vi "Autonomous Independent.vi"   [LabVIEW 2017] (continued)
                  n1161 = call <vilib>:"WPI_RobotDriveTankDrive.vi"("Right axis value"=w3971, "Left axis value"=w3971, "RobotDriveDevRef"=w3970) -> ("RobotDriveDevRef"=w3969:T1)  [unwired: 6 in, 2 out]
                  n1162 = global write "Robot Global Data.vi" "Axes"(w3975) -> ()
                }
                frame #5 {
                  n1163 = global write "Robot Global Data.vi" "Current State"(FALSE ("Current State")) -> ()
                  n1164 = Wait (ms)(milliseconds to wait=u32 400) -> ()  [unwired: 1 out]
                }
                frame #6 {
                  n1165 = global read "Robot Global Data.vi" "Axes"() -> (w3989:dbl[])
                  n1166 = Array To Cluster(array=w3989) -> (cluster=w3988:T15)
                  n1167 = Bundle By Name(cluster=w3988, "Axes[1]"=-1.0) -> (w3991:T15)
                  n1168 = Cluster To Array(cluster=w3991) -> (array=w3990:dbl[])
                  n1169 = global write "Robot Global Data.vi" "Axes"(w3990) -> ()
                }
                frame #7 {
                  n1170 = call "PID Distance.vi"("Distance"=7.0, "Angle"=90.0, "RightEncoder"=w3996, "LeftEncoder"=w3997, "GyroDevRef"=w4002, "RobotDriveDevRef"=w4001) -> ("RightEncoder 2"=w3993:T11, "LeftEncoder 2"=w3994:T11, "GyroDevRef 2"=w3995:T8, "RobotDriveDevRef 2"=w4000:T1)  [unwired: 2 in]
                }
                frame #8 {
                  n1171 = global write "Robot Global Data.vi" "Lift_Position"(1.0) -> ()
                  n1172 = call "PID turning.vi"("Angle"=155.0, "GyroDevRef"=w4008, "RobotDriveDevRef"=w4009) -> ("GyroDevRef 2"=w4004:T8, "RobotDriveDevRef 2"=w4005:T1)  [unwired: 7 in]
                }
                frame #9 {
                  n1173 = global read "Robot Global Data.vi" "PIXY Output"() -> (w4022:T16)
                  n1174 = Unbundle By Name(w4022) -> ("SIGNATURE NUMBER"=w4021:u16)
                  n1175 = global read "Robot Global Data.vi" "Cube Signature"() -> (w4020:dbl)
                  n1176 = Equal?(x=w4021, y=w4020) -> (x = y?=w4019:bool)
                  n1177 = case shown="False" w4019 {
                    tunnel: [w4029 w4033] -> w4011
                    tunnel: [w4028 w4034] -> w4012
                    tunnel: [w4027 w4035] -> w4013
                    tunnel: [w4031 w4036] -> w4014
                    tunnel: w4016 -> [w4028 w4034]
                    tunnel: w4015 -> [w4029 w4033]
                    tunnel: w4017 -> [w4030 w4035]
                    tunnel: w4018 -> [w4032 w4036]
                    frame True {
                      n1178 = call <vilib>:"WPI_GyroGetAngle.vi"("GyroDevRef"=w4030) -> ("Angle"=w4026:dbl, "GyroDevRef"=w4027:T8)  [unwired: 6 in, 3 out]
                      n1179 = In Range and Coerce(upper limit=170.0, x=w4026, lower limit=155.0) -> (coerced(x)=w4025:dbl)  [unwired: 1 out]
                      n1180 = global write "Robot Global Data.vi" "Tracked Angle"(w4025) -> ()
                      n1181 = call "PID vision.vi"("RobotDriveDevRef in"=w4032) -> ("RobotDriveDevRef out"=w4031:T1)  [unwired: 9 in, 1 out]
                    }
                    frame False {
                      n1182 = global write "Robot Global Data.vi" "Tracked Angle"(155.0) -> ()
                    }
                  }
                }
                frame #10 {
                  n1183 = call <vilib>:"WPI_EncoderReset.vi"("EncoderDevRef"=w4044) -> ("EncoderDevRef"=w4039:T11)  [unwired: 9 in, 1 out]
                  n1184 = Wait (ms)(milliseconds to wait=u32 10) -> ()  [unwired: 1 out]
                  n1185 = call <vilib>:"WPI_EncoderReset.vi"("EncoderDevRef"=w4043) -> ("EncoderDevRef"=w4038:T11)  [unwired: 9 in, 1 out]
                }
                frame #11 {
                  n1186 = global write "Robot Global Data.vi" "Lift_Position"(0.0) -> ()
                  n1187 = global read "Robot Global Data.vi" "Axes"() -> (w4059:dbl[])
                  n1188 = Array To Cluster(array=w4059) -> (cluster=w4058:T15)
                  n1189 = global read "Robot Global Data.vi" "Tracked Angle"() -> (w4051:dbl)
                  n1190 = Bundle By Name(cluster=w4058, "Axes[1]"=1.0) -> (w4061:T15)
                  n1191 = call "PID with Infrared.vi"("RobotDriveDevRef"=w4055, "Angle"=w4051, "Encoder Limit"=120.0, "GyroDevRef"=w4053, "Left Encoder"=w4048, "Right Encoder"=w4046, "DigitalInputDevRef"=w4050) -> ("RobotDriveDevRef 2"=w4054:T1, "GyroDevRef 2"=w4052:T8, "Left Encoder 2"=w4047:T11, "Right Encoder 2"=w4045:T11)  [unwired: 4 in, 1 out]
                  n1192 = Cluster To Array(cluster=w4061) -> (array=w4060:dbl[])
                  n1193 = global write "Robot Global Data.vi" "Axes"(w4060) -> ()
                }
                frame #12 {
                  n1194 = global write "Robot Global Data.vi" "Current State"(TRUE ("Current State")) -> ()
                  n1195 = Wait (ms)(milliseconds to wait=u32 750) -> ()  [unwired: 1 out]
                }
                frame #13 {
                  n1196 = case shown="\"R\"" w4068 {
                    tunnel: w4072 -> [w4079 w4143 _]
                    tunnel: w4071 -> [w4074 w4142 _]
                    tunnel: w4070 -> [w4078 w4141 _]
                    tunnel: w4069 -> [w4076 w4140 _]
                    frame "L" {
                      n1197 = flat-sequence {
                        tunnel: [w4084] -> w4077
                        tunnel: w4076 -> [w4083]
                        tunnel: [w4082] -> w4075
                        tunnel: w4074 -> [w4081]
                        tunnel: [w4080] -> w4073
                        tunnel: w4079 -> [w4103]
                        tunnel: w4078 -> [w4102]
                        tunnel: w4077 -> [w4098]
                        tunnel: w4075 -> [w4097]
                        tunnel: w4073 -> [w4096]
                        frame #0 {
                          n1198 = global read "Robot Global Data.vi" "Axes"() -> (w4093:dbl[])
                          n1199 = global write "Robot Global Data.vi" "Lift_Position"(2.0) -> ()
                          n1200 = Wait (ms)(milliseconds to wait=u32 250) -> ()  [unwired: 1 out]
                          n1201 = Array To Cluster(array=w4093) -> (cluster=w4092:T15)
                          n1202 = Bundle By Name(cluster=w4092, "Axes[1]"=-1.0) -> (w4095:T15)
                          n1203 = call <vilib>:"WPI_EncoderGet.vi"("EncoderDevRef"=w4083) -> ("Distance"=w4087:dbl, "EncoderDevRef"=w4082:T11)  [unwired: 5 in, 4 out]
                          n1204 = call <vilib>:"WPI_EncoderGet.vi"("EncoderDevRef"=w4081) -> ("Distance"=w4088:dbl, "EncoderDevRef"=w4080:T11)  [unwired: 5 in, 4 out]
                          n1205 = Add(x=w4087, y=w4088) -> (x+y=w4086:dbl)
                          n1206 = Cluster To Array(cluster=w4095) -> (array=w4094:dbl[])
                          n1207 = global write "Robot Global Data.vi" "Axes"(w4094) -> ()
                          n1208 = Divide(x=w4086, y=2.0) -> (x/y=w4084:dbl)
                        }
                        frame #1 {
                          n1209 = Add(x=w4098, y=15.0 ("Distance")) -> (x+y=w4099:dbl)
                          n1210 = global read "Robot Global Data.vi" "Tracked Angle"() -> (w4101:dbl)
                          n1211 = call "PID Distance.vi"("Distance"=w4099, "Angle"=w4101, "RightEncoder"=w4096, "LeftEncoder"=w4097, "GyroDevRef"=w4102, "RobotDriveDevRef"=w4103) -> ()  [unwired: 2 in, 4 out]
                        }
                        frame #2 {
                          n1212 = global read "Robot Global Data.vi" "Axes"() -> (w4107:dbl[])
                          n1213 = Wait (ms)(milliseconds to wait=u32 200) -> ()  [unwired: 1 out]
                          n1214 = Array To Cluster(array=w4107) -> (cluster=w4106:T15)
                          n1215 = Bundle By Name(cluster=w4106, "Axes[1]"=0.5) -> (w4109:T15)
                          n1216 = Cluster To Array(cluster=w4109) -> (array=w4108:dbl[])
                          n1217 = global write "Robot Global Data.vi" "Axes"(w4108) -> ()
                        }
                        frame #3 {
                          n1218 = global write "Robot Global Data.vi" "Current State"(FALSE ("Current State")) -> ()
                          n1219 = Wait (ms)(milliseconds to wait=u32 500) -> ()  [unwired: 1 out]
                        }
                      }
                    }
                    frame "R" {
                      n1220 = flat-sequence {
                        tunnel: w4143 -> [w4154]
                        tunnel: w4142 -> [w4159]
                        tunnel: w4141 -> [w4153]
                        tunnel: w4140 -> [w4152]
                        tunnel: [w4158] -> w4139
                        tunnel: [w4157] -> w4138
                        tunnel: [w4156] -> w4136
                        tunnel: [w4155] -> w4134
                        tunnel: w4139 -> [w4167]
                        tunnel: w4138 -> [w4166]
                        tunnel: [w4165] -> w4137
                        tunnel: w4136 -> [w4165]
                        tunnel: [w4164] -> w4135
                        tunnel: w4134 -> [w4164]
                        tunnel: [w4163] -> w4132
                        tunnel: [w4162] -> w4130
                        tunnel: w4137 -> [w4174]
                        tunnel: w4135 -> [w4173]
                        tunnel: [w4172] -> w4133
                        tunnel: w4132 -> [w4172]
                        tunnel: [w4171] -> w4131
                        tunnel: w4130 -> [w4171]
                        tunnel: [w4170] -> w4129
                        tunnel: [w4169] -> w4128
                        tunnel: w4133 -> [w4184]
                        tunnel: w4131 -> [w4183]
                        tunnel: w4129 -> [w4182]
                        tunnel: w4128 -> [w4181]
                        tunnel: [w4180] -> w4127
                        tunnel: [w4179] -> w4126
                        tunnel: [w4177] -> w4125
                        tunnel: [w4176] -> w4124
                        tunnel: [w4190] -> w4123
                        tunnel: [w4189] -> w4122
                        tunnel: [w4188] -> w4121
                        tunnel: [w4187] -> w4120
                        tunnel: w4124 -> [w4187]
                        tunnel: w4125 -> [w4188]
                        tunnel: w4126 -> [w4189]
                        tunnel: w4127 -> [w4190]
                        tunnel: [w4200] -> w4113
                        tunnel: w4123 -> [w4200]
                        tunnel: [w4199] -> w4115
                        tunnel: w4122 -> [w4199]
                        tunnel: [w4198] -> w4117
                        tunnel: w4121 -> [w4198]
                        tunnel: [w4197] -> w4119
                        tunnel: w4120 -> [w4197]
                        tunnel: w4119 -> [w4212]
                        tunnel: [w4212] -> w4118
                        tunnel: w4117 -> [w4211]
                        tunnel: [w4211] -> w4116
                        tunnel: w4115 -> [w4210]
                        tunnel: [w4210] -> w4114
                        tunnel: w4113 -> [w4209]
                        tunnel: [w4209] -> w4112
                        tunnel: w4118 -> [w4213]
                        tunnel: w4116 -> [w4214]
                        tunnel: w4114 -> [w4215]
                        tunnel: w4112 -> [w4216]
                        frame #0 {
                          n1221 = global read "Robot Global Data.vi" "Axes"() -> (w4148:dbl[])
                          n1222 = global write "Robot Global Data.vi" "Lift_Position"(2.0) -> ()
                          n1223 = Wait (ms)(milliseconds to wait=u32 250) -> ()  [unwired: 1 out]
                          n1224 = Array To Cluster(array=w4148) -> (cluster=w4147:T15)
                          n1225 = Bundle By Name(cluster=w4147, "Axes[1]"=-1.0) -> (w4150:T15)
                          n1226 = Cluster To Array(cluster=w4150) -> (array=w4149:dbl[])
                          n1227 = global write "Robot Global Data.vi" "Axes"(w4149) -> ()
                        }
                        frame #1 {
                          n1228 = global read "Robot Global Data.vi" "Tracked Angle"() -> (w4151:dbl)
                          n1229 = call "PID Distance.vi"("Distance"=-10.0, "Angle"=w4151, "RightEncoder"=w4159, "LeftEncoder"=w4152, "GyroDevRef"=w4153, "RobotDriveDevRef"=w4154) -> ("RightEncoder 2"=w4155:T11, "LeftEncoder 2"=w4156:T11, "GyroDevRef 2"=w4157:T8, "RobotDriveDevRef 2"=w4158:T1)  [unwired: 2 in]
                        }
                        frame #2 {
                          n1230 = call "PID turning.vi"("Angle"=90.0, "GyroDevRef"=w4166, "RobotDriveDevRef"=w4167) -> ("GyroDevRef 2"=w4162:T8, "RobotDriveDevRef 2"=w4163:T1)  [unwired: 7 in]
                          n1231 = global write "Robot Global Data.vi" "Lift_Position"(3.0) -> ()
                        }
                        frame #3 {
                          n1232 = call <vilib>:"WPI_EncoderReset.vi"("EncoderDevRef"=w4174) -> ("EncoderDevRef"=w4170:T11)  [unwired: 9 in, 1 out]
                          n1233 = Wait (ms)(milliseconds to wait=u32 10) -> ()  [unwired: 1 out]
                          n1234 = call <vilib>:"WPI_EncoderReset.vi"("EncoderDevRef"=w4173) -> ("EncoderDevRef"=w4169:T11)  [unwired: 9 in, 1 out]
                        }
                        frame #4 {
                          n1235 = call "PID Distance.vi"("Distance"=30.0, "Angle"=90.0, "RightEncoder"=w4181, "LeftEncoder"=w4182, "GyroDevRef"=w4183, "RobotDriveDevRef"=w4184) -> ("RightEncoder 2"=w4176:T11, "LeftEncoder 2"=w4177:T11, "GyroDevRef 2"=w4179:T8, "RobotDriveDevRef 2"=w4180:T1)  [unwired: 2 in]
                          n1236 = global write "Robot Global Data.vi" "Lift_Position"(3.0) -> ()
                        }
                        frame #5 {
                          n1237 = global read "Robot Global Data.vi" "Axes"() -> (w4194:dbl[])
                          n1238 = Wait (ms)(milliseconds to wait=u32 500) -> ()  [unwired: 1 out]
                          n1239 = Array To Cluster(array=w4194) -> (cluster=w4193:T15)
                          n1240 = Bundle By Name(cluster=w4193, "Axes[1]"=0.3) -> (w4196:T15)
                          n1241 = Cluster To Array(cluster=w4196) -> (array=w4195:dbl[])
                          n1242 = global write "Robot Global Data.vi" "Axes"(w4195) -> ()
                        }
                        frame #6 {
                          n1243 = global write "Robot Global Data.vi" "Current State"(FALSE ("Current State")) -> ()
                          n1244 = Wait (ms)(milliseconds to wait=u32 400) -> ()  [unwired: 1 out]
                        }
                        frame #7 {
                          n1245 = global read "Robot Global Data.vi" "Axes"() -> (w4206:dbl[])
                          n1246 = Wait (ms)(milliseconds to wait=u32 250) -> ()  [unwired: 1 out]
                          n1247 = Array To Cluster(array=w4206) -> (cluster=w4205:T15)
                          n1248 = Bundle By Name(cluster=w4205, "Axes[1]"=-1.0) -> (w4208:T15)
                          n1249 = Cluster To Array(cluster=w4208) -> (array=w4207:dbl[])
                          n1250 = global write "Robot Global Data.vi" "Axes"(w4207) -> ()
                        }
                        frame #8 {
                          n1251 = call "PID Distance.vi"("Distance"=10.0, "Angle"=90.0, "RightEncoder"=w4213, "LeftEncoder"=w4214, "GyroDevRef"=w4215, "RobotDriveDevRef"=w4216) -> ()  [unwired: 2 in, 4 out]
                        }
                        frame #9 {
                          n1252 = global write "Robot Global Data.vi" "Lift_Position"(1.0) -> ()
                        }
                      }
                    }
                    frame Default {
                    }
                  }
                }
              }
            }
            frame Default {
              n1253 = flat-sequence {
                tunnel: w4221 -> [w4229]
                tunnel: w4220 -> [w4228]
                tunnel: w4222 -> [w4226]
                tunnel: [w4227] -> w4224
                tunnel: w4223 -> [w4225]
                tunnel: w4224 -> [w4232]
                frame #0 {
                  n1254 = call "PID Distance.vi"("Distance"=90.0, "Angle"=0.0, "RightEncoder"=w4225, "LeftEncoder"=w4226, "GyroDevRef"=w4228, "RobotDriveDevRef"=w4229) -> ("RobotDriveDevRef 2"=w4227:T1)  [unwired: 2 in, 3 out]
                }
                frame #1 {
                  w4233 = 0.0
                  n1255 = call <vilib>:"WPI_RobotDriveTankDrive.vi"("Right axis value"=w4233, "Left axis value"=w4233, "RobotDriveDevRef"=w4232) -> ()  [unwired: 6 in, 3 out]
                }
              }
            }
          }
        }
      }
    }
    frame "Left Switch" {
      n1256 = flat-sequence {
        tunnel: w4237 -> [w4256]
        tunnel: w4238 -> [w4262]
        tunnel: w4239 -> [w4261]
        tunnel: [w4260] -> w4243
        tunnel: [w4259] -> w4242
        tunnel: [w4258] -> w4241
        tunnel: [w4257] -> w4240
        tunnel: w4236 -> [w4255]
        tunnel: w4234 -> [w4248]
        tunnel: w4243 -> [w4268]
        tunnel: w4242 -> [w4267]
        tunnel: w4241 -> [w4266]
        tunnel: w4240 -> [w4265]
        tunnel: w4235 -> [w4264]
        frame #0 {
          w4263 = 0.0 ("Left axis value")
          n1257 = global write "Robot Global Data.vi" "Lift_Position"(0.0) -> ()
          n1258 = Multiply(x=w4248, y=1000.0) -> (x*y=w4249:dbl)
          n1259 = global write "Robot Global Data.vi" "Current State"(TRUE ("Current State")) -> ()
          n1260 = global write "Robot Global Data.vi" "Raise_Mast"(FALSE ("Current State")) -> ()
          n1261 = Wait (ms)(milliseconds to wait=10) -> ()  [unwired: 1 out]
          n1262 = Less Or Equal?(x=w4249, y=0.0) -> (x <= y?=w4252:bool)
          n1263 = Greater?(x=w4249, y=11000.0) -> (0:w4251:bool)
          n1264 = call <vilib>:"WPI_EncoderReset.vi"("EncoderDevRef"=w4262) -> ("EncoderDevRef"=w4258:T11)  [unwired: 9 in, 1 out]
          n1265 = call <vilib>:"WPI_EncoderReset.vi"("EncoderDevRef"=w4256) -> ("EncoderDevRef"=w4259:T11)  [unwired: 9 in, 1 out]
          n1266 = Or(x=w4251, y=w4252) -> ()  [unwired: 1 out]
          n1267 = call <vilib>:"WPI_GyroReset.vi"("GyroDevRef"=w4261) -> ("GyroDevRef"=w4257:T8)  [unwired: 9 in, 1 out]
          n1268 = call <vilib>:"WPI_RobotDriveTankDrive.vi"("Right axis value"=w4263, "Left axis value"=w4263, "RobotDriveDevRef"=w4255) -> ("RobotDriveDevRef"=w4260:T1)  [unwired: 6 in, 2 out]
        }
        frame #1 {
          n1269 = case shown="\"L\"" w4264 {
            tunnel: w4268 -> [w4280 w4366 w4488]
            tunnel: w4267 -> [w4277 w4363 w4485]
            tunnel: w4266 -> [w4278 w4364 w4486]
            tunnel: w4265 -> [w4279 w4365 w4487]
            frame "L" {
              n1270 = flat-sequence {
                tunnel: w4280 -> [w4297]
                tunnel: w4277 -> [w4295]
                tunnel: w4278 -> [w4296]
                tunnel: w4279 -> [w4298]
                tunnel: [w4293] -> w4276
                tunnel: [w4292] -> w4274
                tunnel: [w4291] -> w4272
                tunnel: [w4290] -> w4270
                tunnel: w4276 -> [w4308]
                tunnel: [w4304] -> w4275
                tunnel: w4274 -> [w4307]
                tunnel: [w4303] -> w4273
                tunnel: w4272 -> [w4306]
                tunnel: [w4302] -> w4271
                tunnel: w4270 -> [w4305]
                tunnel: [w4301] -> w4269
                tunnel: w4275 -> [w4318]
                tunnel: w4273 -> [w4317]
                tunnel: [w4316] -> w4289
                tunnel: [w4315] -> w4288
                tunnel: [w4314] -> w4287
                tunnel: w4271 -> [w4314]
                tunnel: [w4313] -> w4286
                tunnel: w4269 -> [w4313]
                tunnel: w4289 -> [w4329]
                tunnel: [w4328] -> w4285
                tunnel: w4288 -> [w4334]
                tunnel: [w4334] -> w4284
                tunnel: w4287 -> [w4333]
                tunnel: [w4331] -> w4283
                tunnel: w4286 -> [w4332]
                tunnel: [w4330] -> w4282
                tunnel: w4285 -> [w4339]
                tunnel: [w4338] -> w4281
                tunnel: w4284 -> [w4337]
                tunnel: w4283 -> [w4336]
                tunnel: w4282 -> [w4335]
                tunnel: w4281 -> [w4349]
                frame #0 {
                  n1271 = global write "Robot Global Data.vi" "Raise_Mast"(TRUE ("Current State")) -> ()
                  n1272 = call "PID Distance.vi"("Distance"=60.0, "Angle"=0.0, "RightEncoder"=w4295, "LeftEncoder"=w4296, "GyroDevRef"=w4298, "RobotDriveDevRef"=w4297) -> ("RightEncoder 2"=w4290:T11, "LeftEncoder 2"=w4291:T11, "GyroDevRef 2"=w4292:T8, "RobotDriveDevRef 2"=w4293:T1)  [unwired: 2 in]
                }
                frame #1 {
                  n1273 = global write "Robot Global Data.vi" "Lift_Position"(2.0) -> ()
                  n1274 = call "PID Distance.vi"("Distance"=140.0, "Angle"=0.0, "RightEncoder"=w4305, "LeftEncoder"=w4306, "GyroDevRef"=w4307, "RobotDriveDevRef"=w4308) -> ("RightEncoder 2"=w4301:T11, "LeftEncoder 2"=w4302:T11, "GyroDevRef 2"=w4303:T8, "RobotDriveDevRef 2"=w4304:T1)  [unwired: 2 in]
                  n1275 = Wait (ms)(milliseconds to wait=u32 50) -> ()  [unwired: 1 out]
                }
                frame #2 {
                  n1276 = global read "Robot Global Data.vi" "Axes"() -> (w4321:dbl[])
                  n1277 = call "PID turning.vi"("Angle"=90.0, "GyroDevRef"=w4317, "RobotDriveDevRef"=w4318) -> ("GyroDevRef 2"=w4315:T8, "RobotDriveDevRef 2"=w4316:T1)  [unwired: 7 in]
                  n1278 = global write "Robot Global Data.vi" "Lift_Position"(2.0) -> ()
                  n1279 = Array To Cluster(array=w4321) -> (cluster=w4320:T15)
                  n1280 = Bundle By Name(cluster=w4320, "Axes[1]"=-1.0) -> (w4323:T15)
                  n1281 = Cluster To Array(cluster=w4323) -> (array=w4322:dbl[])
                  n1282 = global write "Robot Global Data.vi" "Axes"(w4322) -> ()
                }
                frame #3 {
                  w4327 = 0.0 ("Left axis value")
                  n1283 = call <vilib>:"WPI_EncoderReset.vi"("EncoderDevRef"=w4333) -> ("EncoderDevRef"=w4331:T11)  [unwired: 9 in, 1 out]
                  n1284 = call <vilib>:"WPI_RobotDriveTankDrive.vi"("Right axis value"=w4327, "Left axis value"=w4327, "RobotDriveDevRef"=w4329) -> ("RobotDriveDevRef"=w4328:T1)  [unwired: 6 in, 2 out]
                  n1285 = Wait (ms)(milliseconds to wait=u32 10) -> ()  [unwired: 1 out]
                  n1286 = call <vilib>:"WPI_EncoderReset.vi"("EncoderDevRef"=w4332) -> ("EncoderDevRef"=w4330:T11)  [unwired: 9 in, 1 out]
                }
                frame #4 {
                  n1287 = call "PID Distance.vi"("Distance"=18.0, "Angle"=90.0, "RightEncoder"=w4335, "LeftEncoder"=w4336, "GyroDevRef"=w4337, "RobotDriveDevRef"=w4339) -> ("RobotDriveDevRef 2"=w4338:T1)  [unwired: 2 in, 3 out]
                }
                frame #5 {
                  w4348 = 0.0 ("Left axis value")
                  n1288 = global read "Robot Global Data.vi" "Axes"() -> (w4344:dbl[])
                  n1289 = call <vilib>:"WPI_RobotDriveTankDrive.vi"("Right axis value"=w4348, "Left axis value"=w4348, "RobotDriveDevRef"=w4349) -> ()  [unwired: 6 in, 3 out]
                  n1290 = Wait (ms)(milliseconds to wait=u32 20) -> ()  [unwired: 1 out]
                  n1291 = Array To Cluster(array=w4344) -> (cluster=w4343:T15)
                  n1292 = Bundle By Name(cluster=w4343, "Axes[1]"=-1.0) -> (w4346:T15)
                  n1293 = Cluster To Array(cluster=w4346) -> (array=w4345:dbl[])
                  n1294 = global write "Robot Global Data.vi" "Axes"(w4345) -> ()
                }
                frame #6 {
                  n1295 = global read "Robot Global Data.vi" "Axes"() -> (w4352:dbl[])
                  n1296 = Wait (ms)(milliseconds to wait=u32 500) -> ()  [unwired: 1 out]
                  n1297 = Array To Cluster(array=w4352) -> (cluster=w4351:T15)
                  n1298 = Bundle By Name(cluster=w4351, "Axes[1]"=1.0) -> (w4354:T15)
                  n1299 = Cluster To Array(cluster=w4354) -> (array=w4353:dbl[])
                  n1300 = global write "Robot Global Data.vi" "Axes"(w4353) -> ()
                }
                frame #7 {
                  n1301 = global write "Robot Global Data.vi" "Current State"(FALSE ("Current State")) -> ()
                  n1302 = Wait (ms)(milliseconds to wait=u32 500) -> ()  [unwired: 1 out]
                }
                frame #8 {
                  n1303 = global read "Robot Global Data.vi" "Axes"() -> (w4359:dbl[])
                  n1304 = Array To Cluster(array=w4359) -> (cluster=w4358:T15)
                  n1305 = Bundle By Name(cluster=w4358, "Axes[1]"=-1.0) -> (w4361:T15)
                  n1306 = Cluster To Array(cluster=w4361) -> (array=w4360:dbl[])
                  n1307 = global write "Robot Global Data.vi" "Axes"(w4360) -> ()
                }
              }
            }
            frame "R" {
              n1308 = flat-sequence {
                tunnel: w4365 -> [w4400]
                tunnel: w4364 -> [w4401]
                tunnel: w4363 -> [w4402]
                tunnel: w4366 -> [w4403]
                tunnel: [w4403] -> w4399
                tunnel: [w4402] -> w4398
                tunnel: [w4401] -> w4397
                tunnel: [w4400] -> w4396
                tunnel: [w4406] -> w4395
                tunnel: [w4407] -> w4394
                tunnel: [w4404] -> w4393
                tunnel: [w4405] -> w4392
                tunnel: w4399 -> [w4410]
                tunnel: w4398 -> [w4408]
                tunnel: w4397 -> [w4409]
                tunnel: w4396 -> [w4411]
                tunnel: w4395 -> [w4418]
                tunnel: w4394 -> [w4417]
                tunnel: [w4421] -> w4391
                tunnel: w4393 -> [w4421]
                tunnel: [w4420] -> w4390
                tunnel: w4392 -> [w4420]
                tunnel: [w4416] -> w4389
                tunnel: [w4415] -> w4388
                tunnel: w4391 -> [w4428]
                tunnel: w4390 -> [w4427]
                tunnel: [w4426] -> w4387
                tunnel: [w4425] -> w4386
                tunnel: [w4424] -> w4385
                tunnel: w4389 -> [w4424]
                tunnel: [w4422] -> w4384
                tunnel: w4388 -> [w4422]
                tunnel: w4387 -> [w4432]
                tunnel: w4386 -> [w4433]
                tunnel: w4385 -> [w4437]
                tunnel: w4384 -> [w4436]
                tunnel: [w4435] -> w4383
                tunnel: [w4434] -> w4382
                tunnel: [w4431] -> w4381
                tunnel: [w4430] -> w4380
                tunnel: [w4448] -> w4379
                tunnel: w4383 -> [w4449]
                tunnel: w4382 -> [w4450]
                tunnel: [w4447] -> w4378
                tunnel: [w4446] -> w4377
                tunnel: w4381 -> [w4446]
                tunnel: [w4445] -> w4376
                tunnel: w4380 -> [w4445]
                tunnel: w4379 -> [w4458]
                tunnel: [w4458] -> w4375
                tunnel: w4378 -> [w4457]
                tunnel: [w4457] -> w4374
                tunnel: [w4454] -> w4373
                tunnel: w4377 -> [w4456]
                tunnel: [w4453] -> w4372
                tunnel: w4376 -> [w4455]
                tunnel: w4375 -> [w4465]
                tunnel: [w4466] -> w4371
                tunnel: w4374 -> [w4464]
                tunnel: w4373 -> [w4463]
                tunnel: w4372 -> [w4462]
                tunnel: [w4461] -> w4370
                tunnel: [w4460] -> w4369
                tunnel: [w4459] -> w4368
                tunnel: [w4469] -> w4367
                tunnel: w4371 -> [w4469]
                tunnel: w4370 -> [_]
                tunnel: w4369 -> [_]
                tunnel: w4368 -> [_]
                tunnel: w4367 -> [w4476]
                frame #0 {
                }
                frame #1 {
                  n1309 = call "PID Distance.vi"("Distance"=220.0, "Angle"=0.0, "RightEncoder"=w4408, "LeftEncoder"=w4409, "GyroDevRef"=w4411, "RobotDriveDevRef"=w4410) -> ("RightEncoder 2"=w4404:T11, "LeftEncoder 2"=w4405:T11, "GyroDevRef 2"=w4407:T8, "RobotDriveDevRef 2"=w4406:T1)  [unwired: 2 in]
                  n1310 = global write "Robot Global Data.vi" "Raise_Mast"(TRUE ("Current State")) -> ()
                }
                frame #2 {
                  n1311 = call "PID turning.vi"("Angle"=90.0, "GyroDevRef"=w4417, "RobotDriveDevRef"=w4418) -> ("GyroDevRef 2"=w4416:T8, "RobotDriveDevRef 2"=w4415:T1)  [unwired: 7 in]
                }
                frame #3 {
                  n1312 = call <vilib>:"WPI_EncoderReset.vi"("EncoderDevRef"=w4427) -> ("EncoderDevRef"=w4425:T11)  [unwired: 9 in, 1 out]
                  n1313 = Wait (ms)(milliseconds to wait=u32 10) -> ()  [unwired: 1 out]
                  n1314 = call <vilib>:"WPI_EncoderReset.vi"("EncoderDevRef"=w4428) -> ("EncoderDevRef"=w4426:T11)  [unwired: 9 in, 1 out]
                }
                frame #4 {
                  n1315 = global read "Robot Global Data.vi" "Axes"() -> (w4441:dbl[])
                  n1316 = global write "Robot Global Data.vi" "Lift_Position"(2.0) -> ()
                  n1317 = call "PID Distance.vi"("Distance"=160.0, "Angle"=90.0, "RightEncoder"=w4432, "LeftEncoder"=w4433, "GyroDevRef"=w4437, "RobotDriveDevRef"=w4436) -> ("RightEncoder 2"=w4430:T11, "LeftEncoder 2"=w4431:T11, "GyroDevRef 2"=w4434:T8, "RobotDriveDevRef 2"=w4435:T1)  [unwired: 2 in]
                  n1318 = Array To Cluster(array=w4441) -> (cluster=w4442:T15)
                  n1319 = Bundle By Name(cluster=w4442, "Axes[1]"=-1.0) -> (w4439:T15)
                  n1320 = Cluster To Array(cluster=w4439) -> (array=w4440:dbl[])
                  n1321 = global write "Robot Global Data.vi" "Axes"(w4440) -> ()
                }
                frame #5 {
                  n1322 = call "PID turning.vi"("Angle"=180.0, "GyroDevRef"=w4450, "RobotDriveDevRef"=w4449) -> ("GyroDevRef 2"=w4447:T8, "RobotDriveDevRef 2"=w4448:T1)  [unwired: 7 in]
                }
                frame #6 {
                  n1323 = call <vilib>:"WPI_EncoderReset.vi"("EncoderDevRef"=w4456) -> ("EncoderDevRef"=w4454:T11)  [unwired: 9 in, 1 out]
                  n1324 = Wait (ms)(milliseconds to wait=u32 10) -> ()  [unwired: 1 out]
                  n1325 = call <vilib>:"WPI_EncoderReset.vi"("EncoderDevRef"=w4455) -> ("EncoderDevRef"=w4453:T11)  [unwired: 9 in, 1 out]
                }
                frame #7 {
                  n1326 = call "PID Distance.vi"("Distance"=20.0, "Angle"=180.0, "RightEncoder"=w4462, "LeftEncoder"=w4463, "GyroDevRef"=w4464, "RobotDriveDevRef"=w4465) -> ("RightEncoder 2"=w4459:T11, "LeftEncoder 2"=w4460:T11, "GyroDevRef 2"=w4461:T8, "RobotDriveDevRef 2"=w4466:T1)  [unwired: 2 in]
                }
                frame #8 {
                  n1327 = global read "Robot Global Data.vi" "Axes"() -> (w4471:dbl[])
                  n1328 = Array To Cluster(array=w4471) -> (cluster=w4470:T15)
                  n1329 = Bundle By Name(cluster=w4470, "Axes[1]"=1.0) -> (w4473:T15)
                  n1330 = Cluster To Array(cluster=w4473) -> (array=w4472:dbl[])
                  n1331 = global write "Robot Global Data.vi" "Axes"(w4472) -> ()
                }
                frame #9 {
                  w4483 = 0.0 ("Left axis value")
                  n1332 = global read "Robot Global Data.vi" "Axes"() -> (w4479:dbl[])
                  n1333 = call <vilib>:"WPI_RobotDriveTankDrive.vi"("Right axis value"=w4483, "Left axis value"=w4483, "RobotDriveDevRef"=w4476) -> ()  [unwired: 6 in, 3 out]
                  n1334 = global write "Robot Global Data.vi" "Lift_Position"(3.0) -> ()
                  n1335 = Wait (ms)(milliseconds to wait=u32 10) -> ()  [unwired: 1 out]
                  n1336 = Array To Cluster(array=w4479) -> (cluster=w4478:T15)
                  n1337 = Bundle By Name(cluster=w4478, "Axes[1]"=1.0) -> (w4481:T15)
                  n1338 = Cluster To Array(cluster=w4481) -> (array=w4480:dbl[])
                  n1339 = global write "Robot Global Data.vi" "Axes"(w4480) -> ()
                }
                frame #10 {
                  n1340 = global write "Robot Global Data.vi" "Current State"(FALSE ("Current State")) -> ()
                }
              }
            }
            frame Default {
              n1341 = flat-sequence {
                tunnel: w4488 -> [w4494]
                tunnel: w4487 -> [w4493]
                tunnel: w4486 -> [w4491]
                tunnel: [w4492] -> w4489
                tunnel: w4485 -> [w4490]
                tunnel: w4489 -> [w4497]
                frame #0 {
                  n1342 = call "PID Distance.vi"("Distance"=90.0, "Angle"=0.0, "RightEncoder"=w4490, "LeftEncoder"=w4491, "GyroDevRef"=w4493, "RobotDriveDevRef"=w4494) -> ("RobotDriveDevRef 2"=w4492:T1)  [unwired: 2 in, 3 out]
                }
                frame #1 {
                  w4498 = 0.0
                  n1343 = call <vilib>:"WPI_RobotDriveTankDrive.vi"("Right axis value"=w4498, "Left axis value"=w4498, "RobotDriveDevRef"=w4497) -> ()  [unwired: 6 in, 3 out]
                }
              }
            }
          }
        }
      }
    }
    frame "Right Scale 1" {
      n1344 = flat-sequence {
        tunnel: w4502 -> [w4534]
        tunnel: w4504 -> [w4532]
        tunnel: w4503 -> [w4531]
        tunnel: w4501 -> [w4530]
        tunnel: [w4529] -> w4509
        tunnel: [w4528] -> w4508
        tunnel: [w4527] -> w4507
        tunnel: [w4526] -> w4506
        tunnel: w4505 -> [w4519]
        tunnel: w4500 -> [w4536]
        tunnel: w4509 -> [w4540]
        tunnel: w4508 -> [w4539]
        tunnel: w4507 -> [w4538]
        tunnel: w4506 -> [w4537]
        tunnel: w4499 -> [w4535]
        frame #0 {
          w4533 = 0.0 ("Left axis value")
          n1345 = global read "Robot Global Data.vi" "Axes"() -> (w4512:dbl[])
          n1346 = Multiply(x=w4519, y=1000.0) -> (x*y=w4520:dbl)
          n1347 = global write "Robot Global Data.vi" "Lift_Position"(0.0) -> ()
          n1348 = global write "Robot Global Data.vi" "Raise_Mast"(FALSE ("Current State")) -> ()
          n1349 = global write "Robot Global Data.vi" "Current State"(TRUE ("Current State")) -> ()
          n1350 = Wait (ms)(milliseconds to wait=10) -> ()  [unwired: 1 out]
          n1351 = Array To Cluster(array=w4512) -> (cluster=w4511:T15)
          n1352 = Bundle By Name(cluster=w4511, "Axes[1]"=-1.0) -> (w4514:T15)
          n1353 = Greater?(x=w4520, y=11000.0) -> (0:w4522:bool)
          n1354 = Equal?(x=w4520, y=0.0) -> (x = y?=w4523:bool)
          n1355 = Or(x=w4522, y=w4523) -> ()  [unwired: 1 out]
          n1356 = Cluster To Array(cluster=w4514) -> (array=w4513:dbl[])
          n1357 = call <vilib>:"WPI_GyroReset.vi"("GyroDevRef"=w4530) -> ("GyroDevRef"=w4526:T8)  [unwired: 9 in, 1 out]
          n1358 = call <vilib>:"WPI_EncoderReset.vi"("EncoderDevRef"=w4532) -> ("EncoderDevRef"=w4528:T11)  [unwired: 9 in, 1 out]
          n1359 = global write "Robot Global Data.vi" "Axes"(w4513) -> ()
          n1360 = call <vilib>:"WPI_EncoderReset.vi"("EncoderDevRef"=w4531) -> ("EncoderDevRef"=w4527:T11)  [unwired: 9 in, 1 out]
          n1361 = call <vilib>:"WPI_RobotDriveTankDrive.vi"("Right axis value"=w4533, "Left axis value"=w4533, "RobotDriveDevRef"=w4534) -> ("RobotDriveDevRef"=w4529:T1)  [unwired: 6 in, 2 out]
        }
        frame #1 {
          n1362 = case shown="\"L\"" w4536 {
            tunnel: w4540 -> [w4544 w4734 w4875]
            tunnel: w4539 -> [w4541 w4731 w4872]
            tunnel: w4538 -> [w4543 w4732 w4873]
            tunnel: w4537 -> [w4542 w4733 w4874]
            tunnel: w4535 -> [w4545 w4730 _]
            frame "L" {
              n1363 = flat-sequence {
                tunnel: w4541 -> [w4607]
                tunnel: w4543 -> [w4608]
                tunnel: w4542 -> [w4609]
                tunnel: w4544 -> [w4610]
                tunnel: [w4603] -> w4601
                tunnel: [w4604] -> w4600
                tunnel: [w4605] -> w4599
                tunnel: [w4606] -> w4598
                tunnel: [w4620] -> w4597
                tunnel: [w4619] -> w4596
                tunnel: [w4617] -> w4595
                tunnel: [w4618] -> w4594
                tunnel: w4601 -> [w4616]
                tunnel: w4600 -> [w4615]
                tunnel: w4599 -> [w4614]
                tunnel: w4598 -> [w4613]
                tunnel: w4597 -> [w4626]
                tunnel: w4596 -> [w4627]
                tunnel: [w4630] -> w4593
                tunnel: w4595 -> [w4630]
                tunnel: [w4629] -> w4592
                tunnel: w4594 -> [w4629]
                tunnel: [w4624] -> w4591
                tunnel: [w4625] -> w4590
                tunnel: w4593 -> [w4637]
                tunnel: w4592 -> [w4636]
                tunnel: [w4635] -> w4589
                tunnel: [w4634] -> w4588
                tunnel: [w4633] -> w4587
                tunnel: w4591 -> [w4633]
                tunnel: [w4631] -> w4586
                tunnel: w4590 -> [w4631]
                tunnel: w4589 -> [w4642]
                tunnel: w4588 -> [w4643]
                tunnel: w4587 -> [w4644]
                tunnel: [w4640] -> w4585
                tunnel: [w4641] -> w4584
                tunnel: w4586 -> [w4645]
                tunnel: [w4638] -> w4583
                tunnel: [w4639] -> w4582
                tunnel: w4585 -> [w4657]
                tunnel: w4584 -> [w4656]
                tunnel: [w4655] -> w4581
                tunnel: [w4654] -> w4580
                tunnel: [w4660] -> w4579
                tunnel: w4583 -> [w4660]
                tunnel: [w4659] -> w4578
                tunnel: w4582 -> [w4659]
                tunnel: w4581 -> [w4666]
                tunnel: [w4666] -> w4577
                tunnel: [w4665] -> w4576
                tunnel: [w4664] -> w4575
                tunnel: [w4663] -> w4574
                tunnel: w4580 -> [w4663]
                tunnel: w4579 -> [w4662]
                tunnel: w4578 -> [w4661]
                tunnel: w4577 -> [w4674]
                tunnel: [w4671] -> w4573
                tunnel: w4576 -> [w4673]
                tunnel: w4575 -> [w4672]
                tunnel: w4574 -> [w4675]
                tunnel: [w4670] -> w4572
                tunnel: [w4669] -> w4571
                tunnel: [w4668] -> w4570
                tunnel: w4573 -> [w4682]
                tunnel: [w4681] -> w4569
                tunnel: w4572 -> [w4679]
                tunnel: [w4678] -> w4568
                tunnel: w4571 -> [w4684]
                tunnel: [w4684] -> w4567
                tunnel: w4570 -> [w4683]
                tunnel: [w4683] -> w4566
                tunnel: w4569 -> [w4695]
                tunnel: [w4689] -> w4565
                tunnel: [w4688] -> w4564
                tunnel: w4568 -> [w4688]
                tunnel: [w4687] -> w4563
                tunnel: w4567 -> [w4687]
                tunnel: [w4686] -> w4562
                tunnel: w4566 -> [w4686]
                tunnel: w4565 -> [w4702]
                tunnel: [w4702] -> w4561
                tunnel: w4564 -> [w4701]
                tunnel: [w4701] -> w4560
                tunnel: w4563 -> [w4700]
                tunnel: [w4700] -> w4559
                tunnel: w4562 -> [w4699]
                tunnel: [w4699] -> w4558
                tunnel: w4561 -> [w4706]
                tunnel: [w4704] -> w4557
                tunnel: w4560 -> [w4705]
                tunnel: [w4703] -> w4556
                tunnel: w4559 -> [w4709]
                tunnel: [w4709] -> w4555
                tunnel: w4558 -> [w4708]
                tunnel: [w4708] -> w4554
                tunnel: w4557 -> [w4722]
                tunnel: w4556 -> [w4721]
                tunnel: w4555 -> [w4720]
                tunnel: w4554 -> [w4719]
                tunnel: [w4713] -> w4553
                tunnel: [w4712] -> w4552
                tunnel: [w4711] -> w4551
                tunnel: [w4710] -> w4550
                tunnel: w4553 -> [w4729]
                tunnel: [w4729] -> w4549
                tunnel: w4552 -> [w4728]
                tunnel: [w4728] -> w4548
                tunnel: w4551 -> [w4727]
                tunnel: [w4727] -> w4547
                tunnel: w4550 -> [w4726]
                tunnel: [w4726] -> w4546
                tunnel: w4549 -> [_]
                tunnel: w4548 -> [_]
                tunnel: w4547 -> [_]
                tunnel: w4546 -> [_]
                tunnel: w4545 -> [_]
                frame #0 {
                  n1364 = global write "Robot Global Data.vi" "Raise_Mast"(FALSE ("Current State")) -> ()
                  n1365 = call "PID Distance.vi"("Distance"=20.0, "Angle"=0.0, "RightEncoder"=w4607, "LeftEncoder"=w4608, "GyroDevRef"=w4609, "RobotDriveDevRef"=w4610) -> ("RightEncoder 2"=w4606:T11, "LeftEncoder 2"=w4605:T11, "GyroDevRef 2"=w4604:T8, "RobotDriveDevRef 2"=w4603:T1)  [unwired: 2 in]
                }
                frame #1 {
                  n1366 = global write "Robot Global Data.vi" "Raise_Mast"(TRUE ("Current State")) -> ()
                  n1367 = call "PID Distance.vi"("Distance"=225.0, "Angle"=0.0, "RightEncoder"=w4613, "LeftEncoder"=w4614, "GyroDevRef"=w4615, "RobotDriveDevRef"=w4616) -> ("RightEncoder 2"=w4617:T11, "LeftEncoder 2"=w4618:T11, "GyroDevRef 2"=w4619:T8, "RobotDriveDevRef 2"=w4620:T1)  [unwired: 2 in]
                }
                frame #2 {
                  n1368 = call "PID turning.vi"("Angle"=-90.0, "GyroDevRef"=w4627, "RobotDriveDevRef"=w4626) -> ("GyroDevRef 2"=w4624:T8, "RobotDriveDevRef 2"=w4625:T1)  [unwired: 7 in]
                }
                frame #3 {
                  n1369 = call <vilib>:"WPI_EncoderReset.vi"("EncoderDevRef"=w4636) -> ("EncoderDevRef"=w4634:T11)  [unwired: 9 in, 1 out]
                  n1370 = Wait (ms)(milliseconds to wait=u32 10) -> ()  [unwired: 1 out]
                  n1371 = call <vilib>:"WPI_EncoderReset.vi"("EncoderDevRef"=w4637) -> ("EncoderDevRef"=w4635:T11)  [unwired: 9 in, 1 out]
                }
                frame #4 {
                  n1372 = global read "Robot Global Data.vi" "Axes"() -> (w4649:dbl[])
                  n1373 = global write "Robot Global Data.vi" "Lift_Position"(2.0) -> ()
                  n1374 = call "PID Distance.vi"("Distance"=199.0, "Angle"=-90.0, "RightEncoder"=w4642, "LeftEncoder"=w4643, "GyroDevRef"=w4644, "RobotDriveDevRef"=w4645) -> ("RightEncoder 2"=w4639:T11, "LeftEncoder 2"=w4638:T11, "GyroDevRef 2"=w4641:T8, "RobotDriveDevRef 2"=w4640:T1)  [unwired: 2 in]
                  n1375 = Array To Cluster(array=w4649) -> (cluster=w4648:T15)
                  n1376 = Bundle By Name(cluster=w4648, "Axes[1]"=-1.0) -> (w4647:T15)
                  n1377 = Cluster To Array(cluster=w4647) -> (array=w4646:dbl[])
                  n1378 = global write "Robot Global Data.vi" "Axes"(w4646) -> ()
                }
                frame #5 {
                  n1379 = call "PID turning.vi"("Angle"=0.0, "GyroDevRef"=w4656, "RobotDriveDevRef"=w4657) -> ("GyroDevRef 2"=w4654:T8, "RobotDriveDevRef 2"=w4655:T1)  [unwired: 7 in]
                }
                frame #6 {
                  n1380 = call <vilib>:"WPI_EncoderReset.vi"("EncoderDevRef"=w4662) -> ("EncoderDevRef"=w4665:T11)  [unwired: 9 in, 1 out]
                  n1381 = call <vilib>:"WPI_EncoderReset.vi"("EncoderDevRef"=w4661) -> ("EncoderDevRef"=w4664:T11)  [unwired: 9 in, 1 out]
                }
                frame #7 {
                  n1382 = call "PID Distance.vi"("Distance"=38.0, "Angle"=0.0, "RightEncoder"=w4672, "LeftEncoder"=w4673, "GyroDevRef"=w4675, "RobotDriveDevRef"=w4674) -> ("RightEncoder 2"=w4668:T11, "LeftEncoder 2"=w4669:T11, "GyroDevRef 2"=w4670:T8, "RobotDriveDevRef 2"=w4671:T1)  [unwired: 2 in]
                  n1383 = global write "Robot Global Data.vi" "Lift_Position"(3.0) -> ()
                }
                frame #8 {
                  n1384 = call "PID turning.vi"("Angle"=20.0, "GyroDevRef"=w4679, "RobotDriveDevRef"=w4682) -> ("GyroDevRef 2"=w4678:T8, "RobotDriveDevRef 2"=w4681:T1)  [unwired: 7 in]
                }
                frame #9 {
                  w4696 = 0.0 ("Left axis value")
                  n1385 = global read "Robot Global Data.vi" "Axes"() -> (w4691:dbl[])
                  n1386 = Wait (ms)(milliseconds to wait=u32 300) -> ()  [unwired: 1 out]
                  n1387 = Array To Cluster(array=w4691) -> (cluster=w4690:T15)
                  n1388 = Bundle By Name(cluster=w4690, "Axes[1]"=0.25) -> (w4693:T15)
                  n1389 = Cluster To Array(cluster=w4693) -> (array=w4692:dbl[])
                  n1390 = call <vilib>:"WPI_RobotDriveTankDrive.vi"("Right axis value"=w4696, "Left axis value"=w4696, "RobotDriveDevRef"=w4695) -> ("RobotDriveDevRef"=w4689:T1)  [unwired: 6 in, 2 out]
                  n1391 = global write "Robot Global Data.vi" "Axes"(w4692) -> ()
                }
                frame #10 {
                  n1392 = global write "Robot Global Data.vi" "Current State"(FALSE ("Current State")) -> ()
                  n1393 = Wait (ms)(milliseconds to wait=u32 400) -> ()  [unwired: 1 out]
                }
                frame #11 {
                  n1394 = call "PID turning.vi"("Angle"=0.0, "GyroDevRef"=w4705, "RobotDriveDevRef"=w4706) -> ("GyroDevRef 2"=w4703:T8, "RobotDriveDevRef 2"=w4704:T1)  [unwired: 7 in]
                }
                frame #12 {
                  n1395 = global read "Robot Global Data.vi" "Axes"() -> (w4718:dbl[])
                  n1396 = Array To Cluster(array=w4718) -> (cluster=w4717:T15)
                  n1397 = call "PID Distance.vi"("Distance"=0.0, "Angle"=0.0, "RightEncoder"=w4719, "LeftEncoder"=w4720, "GyroDevRef"=w4721, "RobotDriveDevRef"=w4722) -> ("RightEncoder 2"=w4710:T11, "LeftEncoder 2"=w4711:T11, "GyroDevRef 2"=w4712:T8, "RobotDriveDevRef 2"=w4713:T1)  [unwired: 2 in]
                  n1398 = Bundle By Name(cluster=w4717, "Axes[1]"=-1.0) -> (w4716:T15)
                  n1399 = Cluster To Array(cluster=w4716) -> (array=w4715:dbl[])
                  n1400 = global write "Robot Global Data.vi" "Axes"(w4715) -> ()
                }
                frame #13 {
                  n1401 = global write "Robot Global Data.vi" "Lift_Position"(1.0) -> ()
                }
                frame #14 {
                }
              }
            }
            frame "R" {
              n1402 = flat-sequence {
                tunnel: [w4782] -> w4774
                tunnel: [w4779] -> w4773
                tunnel: [w4780] -> w4772
                tunnel: [w4781] -> w4771
                tunnel: w4734 -> [w4778]
                tunnel: w4733 -> [w4777]
                tunnel: w4732 -> [w4776]
                tunnel: w4731 -> [w4775]
                tunnel: [w4789] -> w4770
                tunnel: [w4786] -> w4769
                tunnel: [w4787] -> w4768
                tunnel: [w4788] -> w4767
                tunnel: w4774 -> [w4793]
                tunnel: w4773 -> [w4790]
                tunnel: w4772 -> [w4791]
                tunnel: w4771 -> [w4792]
                tunnel: [w4800] -> w4763
                tunnel: [w4799] -> w4764
                tunnel: [w4797] -> w4765
                tunnel: [w4798] -> w4766
                tunnel: w4770 -> [w4804]
                tunnel: w4769 -> [w4801]
                tunnel: w4768 -> [w4802]
                tunnel: w4767 -> [w4803]
                tunnel: [w4812] -> w4762
                tunnel: w4766 -> [w4808]
                tunnel: w4765 -> [w4809]
                tunnel: w4764 -> [w4811]
                tunnel: w4763 -> [w4813]
                tunnel: [w4810] -> w4761
                tunnel: [w4809] -> w4760
                tunnel: [w4808] -> w4759
                tunnel: w4762 -> [w4823]
                tunnel: [w4823] -> w4758
                tunnel: w4761 -> [w4822]
                tunnel: [w4822] -> w4757
                tunnel: [w4821] -> w4756
                tunnel: [w4820] -> w4755
                tunnel: w4760 -> [w4818]
                tunnel: w4759 -> [w4817]
                tunnel: w4758 -> [w4829]
                tunnel: [w4827] -> w4754
                tunnel: w4757 -> [w4828]
                tunnel: [w4826] -> w4753
                tunnel: w4756 -> [w4831]
                tunnel: w4755 -> [w4830]
                tunnel: [w4825] -> w4752
                tunnel: [w4824] -> w4751
                tunnel: w4754 -> [w4838]
                tunnel: [w4837] -> w4750
                tunnel: [w4836] -> w4749
                tunnel: w4753 -> [w4836]
                tunnel: [w4835] -> w4748
                tunnel: w4752 -> [w4835]
                tunnel: [w4834] -> w4747
                tunnel: w4751 -> [w4834]
                tunnel: [w4849] -> w4746
                tunnel: w4750 -> [w4849]
                tunnel: [w4848] -> w4745
                tunnel: w4749 -> [w4848]
                tunnel: [w4847] -> w4744
                tunnel: w4748 -> [w4847]
                tunnel: [w4846] -> w4743
                tunnel: w4747 -> [w4846]
                tunnel: w4746 -> [w4854]
                tunnel: w4745 -> [w4855]
                tunnel: [w4855] -> w4742
                tunnel: [w4854] -> w4741
                tunnel: [w4853] -> w4740
                tunnel: w4744 -> [w4853]
                tunnel: [w4852] -> w4739
                tunnel: w4743 -> [w4852]
                tunnel: [w4868] -> w4738
                tunnel: w4742 -> [w4870]
                tunnel: w4741 -> [w4869]
                tunnel: w4740 -> [w4865]
                tunnel: w4739 -> [w4864]
                tunnel: [w4863] -> w4737
                tunnel: [w4862] -> w4736
                tunnel: [w4861] -> w4735
                tunnel: w4730 -> [_]
                tunnel: w4738 -> [_]
                tunnel: w4737 -> [_]
                tunnel: w4736 -> [_]
                tunnel: w4735 -> [_]
                frame #0 {
                  n1403 = call "PID Distance.vi"("Distance"=20.0, "Angle"=2.0, "RightEncoder"=w4775, "LeftEncoder"=w4776, "GyroDevRef"=w4777, "RobotDriveDevRef"=w4778) -> ("RightEncoder 2"=w4779:T11, "LeftEncoder 2"=w4780:T11, "GyroDevRef 2"=w4781:T8, "RobotDriveDevRef 2"=w4782:T1)  [unwired: 2 in]
                }
                frame #1 {
                  n1404 = call "PID Distance.vi"("Distance"=100.0, "Angle"=2.0, "RightEncoder"=w4790, "LeftEncoder"=w4791, "GyroDevRef"=w4792, "RobotDriveDevRef"=w4793) -> ("RightEncoder 2"=w4786:T11, "LeftEncoder 2"=w4787:T11, "GyroDevRef 2"=w4788:T8, "RobotDriveDevRef 2"=w4789:T1)  [unwired: 2 in]
                  n1405 = global write "Robot Global Data.vi" "Raise_Mast"(TRUE ("Current State")) -> ()
                }
                frame #2 {
                  n1406 = global write "Robot Global Data.vi" "Lift_Position"(2.0) -> ()
                  n1407 = call "PID Distance.vi"("Distance"=300.0, "Angle"=2.0, "RightEncoder"=w4801, "LeftEncoder"=w4802, "GyroDevRef"=w4803, "RobotDriveDevRef"=w4804) -> ("RightEncoder 2"=w4797:T11, "LeftEncoder 2"=w4798:T11, "GyroDevRef 2"=w4799:T8, "RobotDriveDevRef 2"=w4800:T1)  [unwired: 2 in]
                  n1408 = global write "Robot Global Data.vi" "Raise_Mast"(TRUE ("Current State")) -> ()
                }
                frame #3 {
                  n1409 = global write "Robot Global Data.vi" "Lift_Position"(3.0) -> ()
                  n1410 = call "PID turning.vi"("Angle"=-90.0, "GyroDevRef"=w4811, "RobotDriveDevRef"=w4813) -> ("GyroDevRef 2"=w4810:T8, "RobotDriveDevRef 2"=w4812:T1)  [unwired: 7 in]
                  n1411 = global write "Robot Global Data.vi" "Raise_Mast"(TRUE ("Current State")) -> ()
                }
                frame #4 {
                  n1412 = call <vilib>:"WPI_EncoderReset.vi"("EncoderDevRef"=w4817) -> ("EncoderDevRef"=w4820:T11)  [unwired: 9 in, 1 out]
                  n1413 = Wait (ms)(milliseconds to wait=u32 10) -> ()  [unwired: 1 out]
                  n1414 = call <vilib>:"WPI_EncoderReset.vi"("EncoderDevRef"=w4818) -> ("EncoderDevRef"=w4821:T11)  [unwired: 9 in, 1 out]
                }
                frame #5 {
                  n1415 = call "PID Distance.vi"("Distance"=25.0, "Angle"=-90.0, "RightEncoder"=w4831, "LeftEncoder"=w4830, "GyroDevRef"=w4828, "RobotDriveDevRef"=w4829) -> ("RightEncoder 2"=w4824:T11, "LeftEncoder 2"=w4825:T11, "GyroDevRef 2"=w4826:T8, "RobotDriveDevRef 2"=w4827:T1)  [unwired: 2 in]
                }
                frame #6 {
                  w4839 = 0.0 ("Left axis value")
                  n1416 = global read "Robot Global Data.vi" "Axes"() -> (w4842:dbl[])
                  n1417 = Wait (ms)(milliseconds to wait=u32 500) -> ()  [unwired: 1 out]
                  n1418 = Array To Cluster(array=w4842) -> (cluster=w4841:T15)
                  n1419 = Bundle By Name(cluster=w4841, "Axes[1]"=0.25) -> (w4844:T15)
                  n1420 = Cluster To Array(cluster=w4844) -> (array=w4843:dbl[])
                  n1421 = call <vilib>:"WPI_RobotDriveTankDrive.vi"("Right axis value"=w4839, "Left axis value"=w4839, "RobotDriveDevRef"=w4838) -> ("RobotDriveDevRef"=w4837:T1)  [unwired: 6 in, 2 out]
                  n1422 = global write "Robot Global Data.vi" "Axes"(w4843) -> ()
                }
                frame #7 {
                  n1423 = global write "Robot Global Data.vi" "Current State"(FALSE ("Current State")) -> ()
                  n1424 = Wait (ms)(milliseconds to wait=u32 400) -> ()  [unwired: 1 out]
                }
                frame #8 {
                  n1425 = global read "Robot Global Data.vi" "Axes"() -> (w4857:dbl[])
                  n1426 = Array To Cluster(array=w4857) -> (cluster=w4856:T15)
                  n1427 = Bundle By Name(cluster=w4856, "Axes[1]"=-1.0) -> (w4859:T15)
                  n1428 = Cluster To Array(cluster=w4859) -> (array=w4858:dbl[])
                  n1429 = global write "Robot Global Data.vi" "Axes"(w4858) -> ()
                }
                frame #9 {
                  n1430 = call "PID Distance.vi"("Distance"=0.0, "Angle"=-90.0, "RightEncoder"=w4864, "LeftEncoder"=w4865, "GyroDevRef"=w4870, "RobotDriveDevRef"=w4869) -> ("RightEncoder 2"=w4861:T11, "LeftEncoder 2"=w4862:T11, "GyroDevRef 2"=w4863:T8, "RobotDriveDevRef 2"=w4868:T1)  [unwired: 2 in]
                }
                frame #10 {
                  n1431 = global write "Robot Global Data.vi" "Lift_Position"(1.0) -> ()
                }
              }
            }
            frame Default {
              n1432 = flat-sequence {
                tunnel: w4875 -> [w4881]
                tunnel: w4874 -> [w4880]
                tunnel: w4873 -> [w4878]
                tunnel: [w4879] -> w4876
                tunnel: w4872 -> [w4877]
                tunnel: w4876 -> [w4884]
                frame #0 {
                  n1433 = call "PID Distance.vi"("Distance"=90.0, "Angle"=0.0, "RightEncoder"=w4877, "LeftEncoder"=w4878, "GyroDevRef"=w4880, "RobotDriveDevRef"=w4881) -> ("RobotDriveDevRef 2"=w4879:T1)  [unwired: 2 in, 3 out]
                }
                frame #1 {
                  w4885 = 0.0
                  n1434 = call <vilib>:"WPI_RobotDriveTankDrive.vi"("Right axis value"=w4885, "Left axis value"=w4885, "RobotDriveDevRef"=w4884) -> ()  [unwired: 6 in, 3 out]
                }
              }
            }
          }
        }
      }
    }
    frame "Right Scale C" {
      n1435 = flat-sequence {
        tunnel: w4892 -> [w4921]
        tunnel: w4889 -> [w4919]
        tunnel: w4890 -> [w4918]
        tunnel: w4891 -> [w4917]
        tunnel: [w4916] -> w4896
        tunnel: [w4915] -> w4895
        tunnel: [w4914] -> w4894
        tunnel: [w4913] -> w4893
        tunnel: w4888 -> [w4906]
        tunnel: w4887 -> [w4923]
        tunnel: w4896 -> [w4927]
        tunnel: w4895 -> [w4926]
        tunnel: w4894 -> [w4925]
        tunnel: w4893 -> [w4924]
        tunnel: w4886 -> [w4922]
        frame #0 {
          w4920 = 0.0 ("Left axis value")
          n1436 = global read "Robot Global Data.vi" "Axes"() -> (w4899:dbl[])
          n1437 = Multiply(x=w4906, y=1000.0) -> (x*y=w4907:dbl)
          n1438 = global write "Robot Global Data.vi" "Lift_Position"(0.0) -> ()
          n1439 = global write "Robot Global Data.vi" "Raise_Mast"(FALSE ("Current State")) -> ()
          n1440 = global write "Robot Global Data.vi" "Current State"(TRUE ("Current State")) -> ()
          n1441 = Wait (ms)(milliseconds to wait=10) -> ()  [unwired: 1 out]
          n1442 = Array To Cluster(array=w4899) -> (cluster=w4898:T15)
          n1443 = Bundle By Name(cluster=w4898, "Axes[1]"=-1.0) -> (w4901:T15)
          n1444 = Greater?(x=w4907, y=11000.0) -> (0:w4909:bool)
          n1445 = Equal?(x=w4907, y=0.0) -> (x = y?=w4910:bool)
          n1446 = Or(x=w4909, y=w4910) -> ()  [unwired: 1 out]
          n1447 = Cluster To Array(cluster=w4901) -> (array=w4900:dbl[])
          n1448 = call <vilib>:"WPI_GyroReset.vi"("GyroDevRef"=w4917) -> ("GyroDevRef"=w4913:T8)  [unwired: 9 in, 1 out]
          n1449 = call <vilib>:"WPI_EncoderReset.vi"("EncoderDevRef"=w4919) -> ("EncoderDevRef"=w4915:T11)  [unwired: 9 in, 1 out]
          n1450 = global write "Robot Global Data.vi" "Axes"(w4900) -> ()
          n1451 = call <vilib>:"WPI_EncoderReset.vi"("EncoderDevRef"=w4918) -> ("EncoderDevRef"=w4914:T11)  [unwired: 9 in, 1 out]
          n1452 = call <vilib>:"WPI_RobotDriveTankDrive.vi"("Right axis value"=w4920, "Left axis value"=w4920, "RobotDriveDevRef"=w4921) -> ("RobotDriveDevRef"=w4916:T1)  [unwired: 6 in, 2 out]
        }
        frame #1 {
          n1453 = case shown="\"R\"" w4923 {
            tunnel: w4927 -> [w4931 w5001 w5142]
            tunnel: w4926 -> [w4928 w4998 w5139]
            tunnel: w4925 -> [w4930 w4999 w5140]
            tunnel: w4924 -> [w4929 w5000 w5141]
            tunnel: w4922 -> [w4932 w4997 _]
            frame "L" {
              n1454 = flat-sequence {
                tunnel: w4928 -> [w4954]
                tunnel: w4930 -> [w4955]
                tunnel: w4929 -> [w4956]
                tunnel: w4931 -> [w4957]
                tunnel: [w4950] -> w4948
                tunnel: [w4951] -> w4947
                tunnel: [w4952] -> w4946
                tunnel: [w4953] -> w4945
                tunnel: [w4967] -> w4944
                tunnel: [w4966] -> w4943
                tunnel: [w4964] -> w4942
                tunnel: [w4965] -> w4941
                tunnel: w4948 -> [w4963]
                tunnel: w4947 -> [w4962]
                tunnel: w4946 -> [w4961]
                tunnel: w4945 -> [w4960]
                tunnel: w4944 -> [w4973]
                tunnel: w4943 -> [w4974]
                tunnel: [w4977] -> w4940
                tunnel: w4942 -> [w4977]
                tunnel: [w4976] -> w4939
                tunnel: w4941 -> [w4976]
                tunnel: [w4971] -> w4938
                tunnel: [w4972] -> w4937
                tunnel: w4940 -> [w4984]
                tunnel: w4939 -> [w4983]
                tunnel: [w4982] -> w4936
                tunnel: [w4981] -> w4935
                tunnel: [w4980] -> w4934
                tunnel: w4938 -> [w4980]
                tunnel: [w4978] -> w4933
                tunnel: w4937 -> [w4978]
                tunnel: w4932 -> [_]
                tunnel: w4933 -> [w4988]
                tunnel: w4934 -> [w4987]
                tunnel: w4935 -> [w4986]
                tunnel: w4936 -> [w4985]
                frame #0 {
                  n1455 = global write "Robot Global Data.vi" "Raise_Mast"(FALSE ("Current State")) -> ()
                  n1456 = call "PID Distance.vi"("Distance"=20.0, "Angle"=0.0, "RightEncoder"=w4954, "LeftEncoder"=w4955, "GyroDevRef"=w4956, "RobotDriveDevRef"=w4957) -> ("RightEncoder 2"=w4953:T11, "LeftEncoder 2"=w4952:T11, "GyroDevRef 2"=w4951:T8, "RobotDriveDevRef 2"=w4950:T1)  [unwired: 2 in]
                }
                frame #1 {
                  n1457 = global write "Robot Global Data.vi" "Raise_Mast"(TRUE ("Current State")) -> ()
                  n1458 = call "PID Distance.vi"("Distance"=225.0, "Angle"=0.0, "RightEncoder"=w4960, "LeftEncoder"=w4961, "GyroDevRef"=w4962, "RobotDriveDevRef"=w4963) -> ("RightEncoder 2"=w4964:T11, "LeftEncoder 2"=w4965:T11, "GyroDevRef 2"=w4966:T8, "RobotDriveDevRef 2"=w4967:T1)  [unwired: 2 in]
                }
                frame #2 {
                  n1459 = call "PID turning.vi"("Angle"=-90.0, "GyroDevRef"=w4974, "RobotDriveDevRef"=w4973) -> ("GyroDevRef 2"=w4971:T8, "RobotDriveDevRef 2"=w4972:T1)  [unwired: 7 in]
                }
                frame #3 {
                  n1460 = call <vilib>:"WPI_EncoderReset.vi"("EncoderDevRef"=w4983) -> ("EncoderDevRef"=w4981:T11)  [unwired: 9 in, 1 out]
                  n1461 = Wait (ms)(milliseconds to wait=u32 10) -> ()  [unwired: 1 out]
                  n1462 = call <vilib>:"WPI_EncoderReset.vi"("EncoderDevRef"=w4984) -> ("EncoderDevRef"=w4982:T11)  [unwired: 9 in, 1 out]
                }
                frame #4 {
                  n1463 = global read "Robot Global Data.vi" "Axes"() -> (w4992:dbl[])
                  n1464 = global write "Robot Global Data.vi" "Lift_Position"(2.0) -> ()
                  n1465 = call "PID Distance.vi"("Distance"=100.0, "Angle"=-90.0, "RightEncoder"=w4985, "LeftEncoder"=w4986, "GyroDevRef"=w4987, "RobotDriveDevRef"=w4988) -> ()  [unwired: 2 in, 4 out]
                  n1466 = Array To Cluster(array=w4992) -> (cluster=w4991:T15)
                  n1467 = Bundle By Name(cluster=w4991, "Axes[1]"=-1.0) -> (w4990:T15)
                  n1468 = Cluster To Array(cluster=w4990) -> (array=w4989:dbl[])
                  n1469 = global write "Robot Global Data.vi" "Axes"(w4989) -> ()
                }
              }
            }
            frame "R" {
              n1470 = flat-sequence {
                tunnel: [w5049] -> w5041
                tunnel: [w5046] -> w5040
                tunnel: [w5047] -> w5039
                tunnel: [w5048] -> w5038
                tunnel: w5001 -> [w5045]
                tunnel: w5000 -> [w5044]
                tunnel: w4999 -> [w5043]
                tunnel: w4998 -> [w5042]
                tunnel: [w5056] -> w5037
                tunnel: [w5053] -> w5036
                tunnel: [w5054] -> w5035
                tunnel: [w5055] -> w5034
                tunnel: w5041 -> [w5060]
                tunnel: w5040 -> [w5057]
